vi "zmq poll.vi"(8 "error in (no error)":errorcluster, 9 "timeout_":i32, 10 "nitems_":i32, 11 "items_":T1) -> (0 "error out":errorcluster, 2 "function return":i32, 3 "items_ out":T1)   [LabVIEW 2025, in "libzmq-v143-mt-4_3_6.lvlib"]
doc: "ZMQ_EXPORT int zmq_poll (zmq_pollitem_t *items_, int nitems_, long timeout_);"
uses:
  libzmq-v143-mt-4_3_6.lvlib
  LV/LibZMQ/libzmq/lv_x86/bin/Release/libzmq-v143-mt-4_3_6.dll
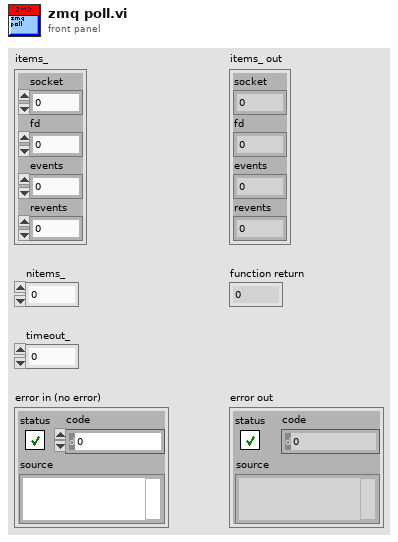
[diagram p1: front panel]
types:
  T1 = cluster{"socket":u32, "fd":i32, "events":i16, "revents":i16}
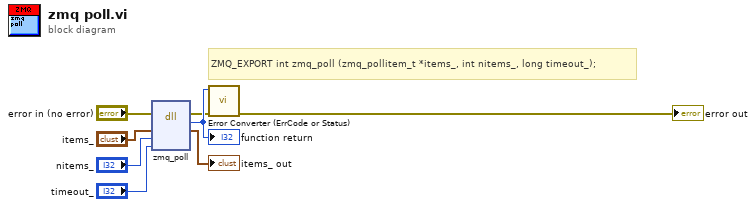
[diagram p0: block diagram]
diagram:
  # "ZMQ_EXPORT int zmq_poll (zmq_pollitem_t *items_, int nitems_, long timeout_);"
  n1 = dll-call lib="C:/LV/LibZMQ/libzmq/lv_x86/bin/Release/libzmq-v143-mt-4_3_6.*" fn="zmq_poll"(error in="error in (no error)", "items_"="items_", "nitems_"="nitems_", "timeout_"="timeout_") -> (error out=w2:errorcluster, w8:i32, "items_"=→"items_ out":T1)  [unwired: 4 in, 1 out]
  "function return" <- w8
  n2 = call "Error Converter (ErrCode or Status).vi"("error in (no error)"=w2, "error code"=w8) -> ("error out"=→"error out":errorcluster)  [unwired: 9 in]
